vi "Array checker.vi"() -> ()   [LabVIEW 2018]
panel:
  out "sorted array":dbl[](array[numeric])
  in  "Array":dbl[](array[numeric])
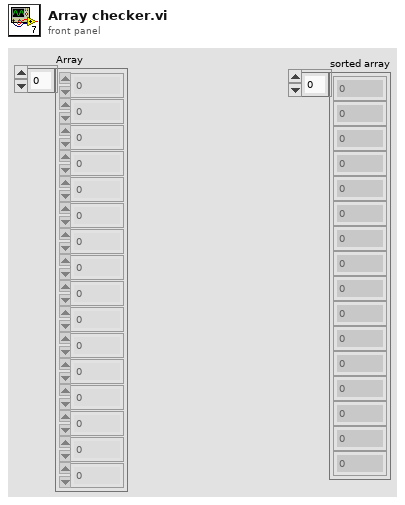
[diagram p1: front panel]
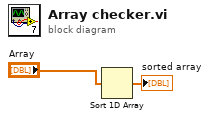
[diagram p0: block diagram]
diagram:
  n1 = Sort 1D Array(array="Array") -> (sorted array=→"sorted array":dbl[])
